vi "SP Check Segmented Limit (single X Y).vi"(0 "Single Segment":cluster{"X":dbl[], "Y":dbl[]} {"Y" format="%0.2f"; "X" format="%0.2f"}, 1 "x0":dbl format="%0.2f", 2 "dx":dbl format="%0.2f", 3 "error in":errorcluster) -> (8 "limit spec ok":bool, 10 "error out":errorcluster)   [LabVIEW 2011]
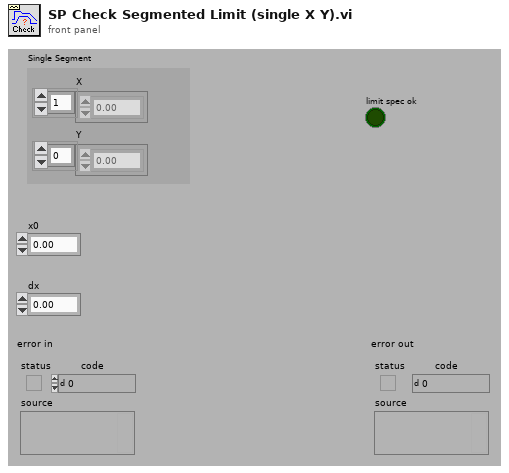
[diagram p1: front panel]
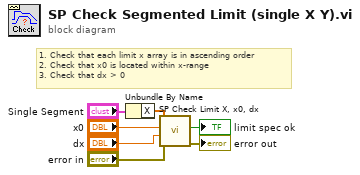
[diagram p0: block diagram]
diagram:
  # "1. Check that each limit x array is in ascending order\n2. Check that x0 is located within x-range\n3. Check that dx > 0"
  n1 = Unbundle By Name("Single Segment") -> ("X"=w6:dbl[])
  n2 = call "SP Check Limit X, x0, dx.vi"("X"=w6, "x0"="x0", "dX"="dx", "error in"="error in") -> ("Limit Spec OK"=→"limit spec ok":bool, "error out"=→"error out":errorcluster)  [unwired: 1 in, 4 out]
